vi "HandleItemActivation.vi"(8 "error in (no error)":errorcluster, 11 "GettingStartedWindow.lvlib:Manual.lvclass":refnum<class "Manual.lvclass">) -> (0 "error out":errorcluster, 3 "GettingStartedWindow.lvlib:Manual.lvclass 2":refnum<class "Manual.lvclass">)   [LabVIEW 2009, in "NavScreen.lvlib" / "Manual.lvclass"]
uses:
  Manual.lvclass
  Manual.lvclass/Manual.ctl
  <vilib>/Platform/browser.llb/Open Acrobat Document.vi
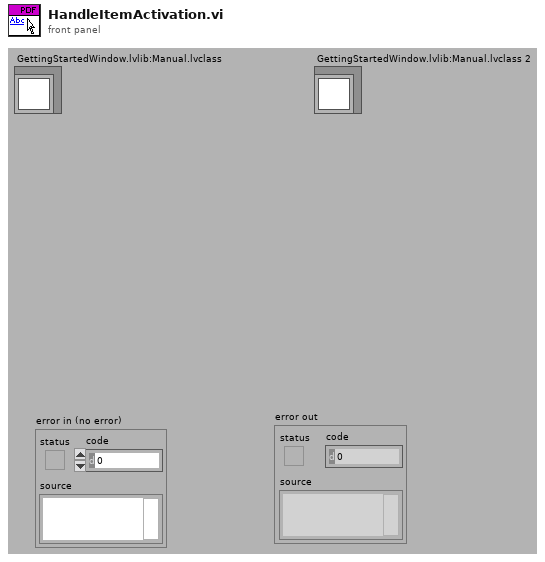
[diagram p1: front panel]
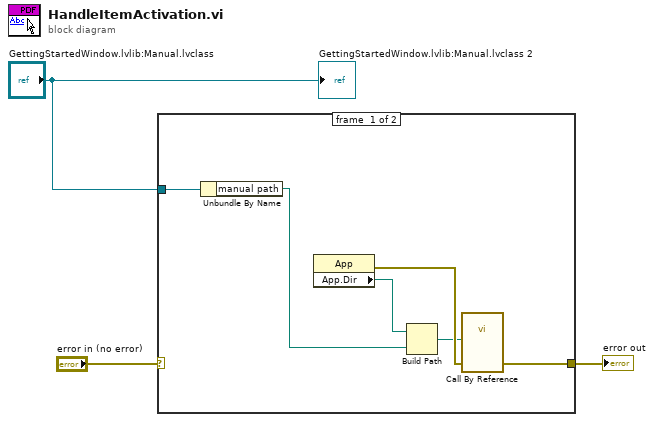
[diagram p0: block diagram]
diagram:
  n1 = case shown="No Error" "error in (no error)" {
    selector: "error in (no error)" -> [_ w10]
    tunnel: [w9 w10] -> w2
    tunnel: "GettingStartedWindow.lvlib:Manual.lvclass" -> [w6 _]
    frame #0 {
      n2 = Unbundle By Name(w6) -> ("manual path"=w5:path)
      n3 = property class="App"() -> (error out=w7:errorcluster, "App.Dir"=w8:path)  [unwired: 2 in, 1 out]
      n4 = Build Path(base path=w8, name or relative path=w5) -> (appended path=w4:path)
      n5 = call-by-ref "?"("error in (no error)"=w7, "acrobat document"=w4) -> ("error out"=w9:errorcluster)  [unwired: 7 in, 2 out]
    }
    frame #1 {
    }
  }
  "error out" <- w2
  "GettingStartedWindow.lvlib:Manual.lvclass 2" <- "GettingStartedWindow.lvlib:Manual.lvclass"
